vi "Render Section-Text.vi"(8 "Error In":errorcluster) -> (0 "Error Out":errorcluster)   [LabVIEW 2018, in "Tests.lvlib" / "Render.lvlib"]
uses:
  Render.lvlib
  src/Toolkit/Data/Array/Array.lvclass
  D:/Users/cfield/Code/Field R&D Services/Labstache/src/Toolkit/Data/Datum/Datum.lvclass
  src/Toolkit/Data/Map/Map.lvclass
  src/Toolkit/Data/Array/Support/From Mapped Strings.vi
  src/Toolkit/Data/Map/Support/From Datum.vi
  src/Toolkit/Low-Level/Renderer/Renderer.lvclass
  <vilib>/addons/_JKI Toolkits/Caraya/classes/Test/Test.lvclass
  <vilib>/addons/_JKI Toolkits/Caraya/classes/Assert/Assert.lvclass
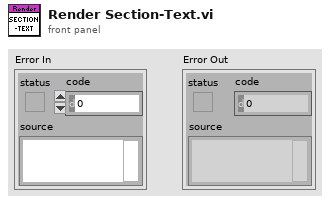
[diagram p1: front panel]
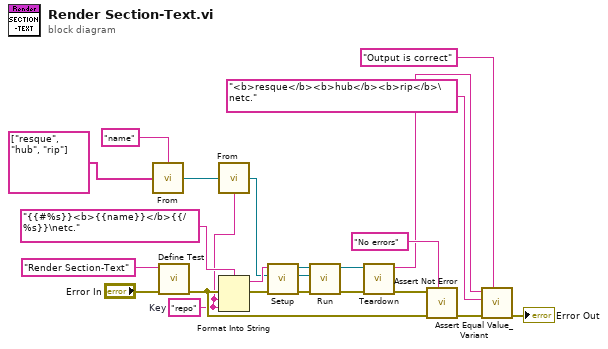
[diagram p0: block diagram]
diagram:
  w7 = "repo"  # Key
  n1 = call-poly "From.vi"("Strings"=string[] ["resque", "hub", "rip"], "Key"="name") -> ("Array"=w8:refnum<class "Array.lvclass">)
  n2 = call <vilib>:"Define Test.vi"("error in (no error)"="Error In", "Label (VI Title)"="Render Section-Text") -> ("error out"=w12:errorcluster)  [unwired: 9 in]
  n3 = call-poly "From.vi"("Value"=w8, "Key"=w7) -> ("Map"=w2:refnum<class "Map.lvclass">)
  n4 = Format Into String(format string="{{#%s}}<b>{{name}}</b>{{/%s}}\netc.", error in=w12, w7, w7) -> (resulting string=w9:string, error out=w11:errorcluster)  [unwired: 1 in]
  n5 = call "Setup.vi"("Error In"=w11, "Data"=w2, "Value"=w9) -> ("Error Out"=w13:errorcluster, "Abstract Syntax Tree"=w1:refnum<class "Root.lvclass">, "Renderer"=w14:refnum<class "Renderer.lvclass">)  [unwired: 6 in]
  n6 = call-dynamic "Run.vi"("Error In"=w13, "Abstract Syntax Tree"=w1, "Renderer In"=w14) -> ("Error Out"=w15:errorcluster, "Renderer Out"=w3:refnum<class "Renderer.lvclass">)  [unwired: 7 in]
  n7 = call "Teardown.vi"("Error In"=w15, "Renderer"=w3) -> ("Error Out"=w17:errorcluster, "Output"=w16:string)  [unwired: 8 in]
  n8 = call <vilib>:"Assert Not Error.vi"("Label"="No errors", "error in (no error)"=w12, "Not Error?"=w17) -> ("error out"=w20:errorcluster)  [unwired: 8 in]
  n9 = call <vilib>:"Assert Equal Value_Variant.vi"("Label"="Output is correct", "error in (no error)"=w20, "Y"="<b>resque</b><b>hub</b><b>rip</b>\netc.", "X"=w16) -> ("error out"=→"Error Out":errorcluster)  [unwired: 7 in]
